vi "DB Tools Move To Previous Record.vi"   [LabVIEW 2013, in "NI_Database_API_64.lvlib"]
doc: "Moves the cursor to point to the previous record in the recordset. You cannot use this VI with a forward-only cursor. Wire data to the reference input to determine the polymorphic instance to use or manually select the instance."
uses:
  NI_Database_API_64.lvlib
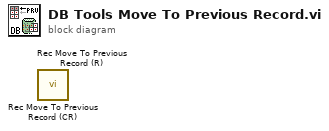
[diagram p0: block diagram]
diagram:
  n1 = call "Rec Move To Previous Record (CR).vi"() -> ()  [unwired: 10 in, 2 out]
  n2 = call "Rec Move To Previous Record (R).vi"() -> ()  [unwired: 10 in, 2 out]
